vi "Decimals Format String.vi"(4 "Decimals":u8, 5 "Suffix (None)":string) -> (7 "Format String":string)   [LabVIEW 2020, in "VolatusGUIEditorCore.lvlib"]
uses:
  VolatusGUIEditorCore.lvlib
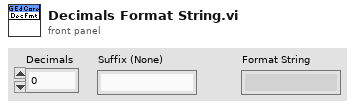
[diagram p1: front panel]
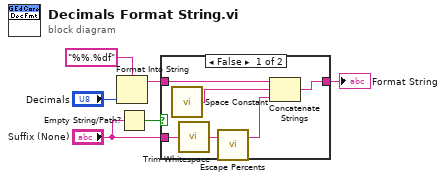
[diagram p0: block diagram]
diagram:
  n1 = Format Into String(format string="%%.%df", "Decimals") -> (resulting string=w2:string)  [unwired: 2 in, 1 out]
  n2 = Empty String/Path?(string/path="Suffix (None)") -> (empty?=w4:bool)
  n3 = case shown="False" w4 {
    tunnel: "Suffix (None)" -> [w12 _]
    tunnel: w2 -> [w11 w13]
    tunnel: [w9 w13] -> w1
    frame False {
      n4 = call <vilib>:"Space Constant.vi"() -> ("String"=w10:string)
      n5 = call <vilib>:"Trim Whitespace.vi"("string"=w12) -> ("trimmed string"=w8:string)  [unwired: 1 in]
      n6 = call "Escape Percents.vi"("String in"=w8) -> ("String"=w7:string)  [unwired: 6 in]
      n7 = Concatenate Strings(w11, w10, w7) -> (w9:string)
    }
    frame True {
    }
  }
  "Format String" <- w1
